vi "Database Query Search.vi"(8 "error in (no error)":errorcluster, 10 "SQL query":string, 11 "Database in":refnum<class "DatabaseAPI.lvclass">) -> (0 "error out":errorcluster, 3 "Database out":refnum<class "DatabaseAPI.lvclass">)   [LabVIEW 2015, in "DatabaseAPI.lvclass"]
uses:
  DatabaseAPI.lvclass
  DatabaseAPI.lvclass/DatabaseAPI.ctl
  <vilib>/addons/database/Connection.llb/DB Tools Open Connec (String).vi
  <vilib>/addons/database/Connection.llb/Conn Execute.vi
  <vilib>/addons/database/Recordset.llb/Rec Destroy - Connection.vi
  <vilib>/addons/database/NI_Database_API.lvlib
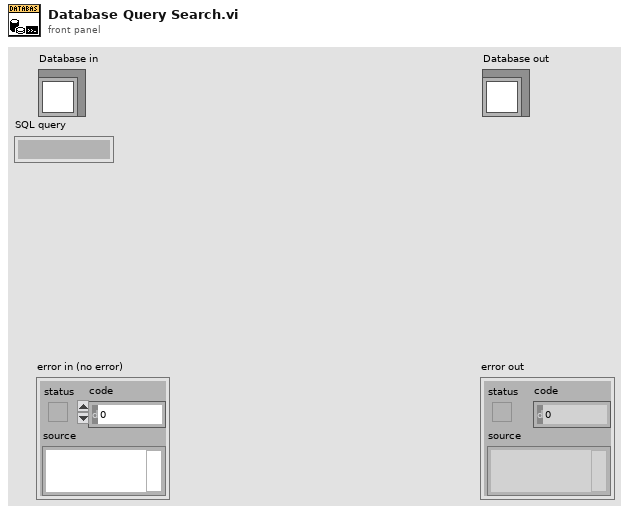
[diagram p1: front panel]
types:
  T1 = typedef "NI_Database_API.lvlib/Conn ObjectReference.ctl" = refnum<k1>
  T2 = typedef "NI_Database_API.lvlib/Rec ObjectReference.ctl" = refnum<k1>
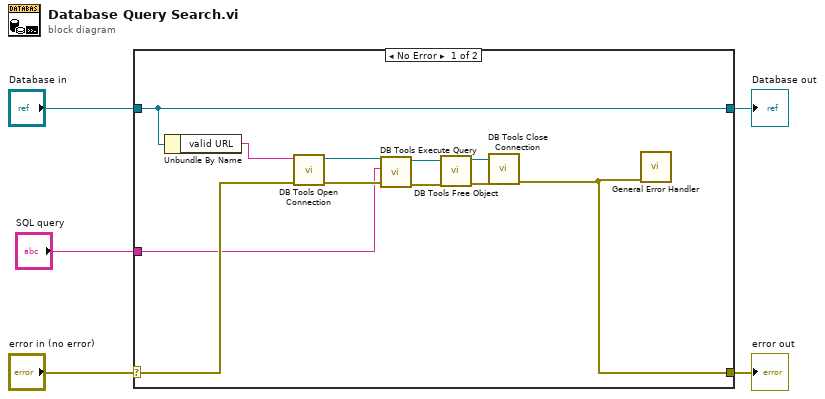
[diagram p0: block diagram]
diagram:
  n1 = case shown="No Error" "error in (no error)" {
    selector: "error in (no error)" -> [w12 w18]
    tunnel: [w6 w18] -> w4
    tunnel: [w16 w17] -> w2
    tunnel: "Database in" -> [w16 w17]
    tunnel: "SQL query" -> [w11 _]
    frame No Error {
      n2 = Unbundle By Name(w16) -> ("valid URL"=w15:string)
      n3 = call-poly <vilib>:"DB Tools Open Connection.vi"("error in (no error)"=w12, "connection information"=w15) -> ("error out"=w13:errorcluster, "connection reference"=w14:T1)  [unwired: 6 in]
      n4 = call-poly <vilib>:"DB Tools Execute Query.vi"("error in (no error)"=w13, "SQL query"=w11, "connection reference"=w14) -> ("error out"=w9:errorcluster, "recordset reference"=w10:T2)  [unwired: 5 in]
      n5 = call-poly <vilib>:"DB Tools Free Object.vi"("error in (no error)"=w9, "recordset reference"=w10) -> ("error out"=w7:errorcluster, "connection reference"=w8:T1)  [unwired: 8 in]
      n6 = call <vilib>:"DB Tools Close Connection.vi"("error in (no error)"=w7, "connection reference"=w8) -> ("error out"=w6:errorcluster)  [unwired: 5 in]
      n7 = call <vilib>:"General Error Handler.vi"("error in (no error)"=w6) -> ()  [unwired: 10 in, 5 out]
    }
    frame Error {
    }
  }
  "error out" <- w4
  "Database out" <- w2
